vi "format_arcmin2arcsecstr.vi"(5 "RA arcmin":dbl, 9 "DEC Arcmin":dbl) -> (4 "Formatted RA":string, 8 "Formatted Dist":string, 15 "Formatted DEC":string)   [LabVIEW 2019]
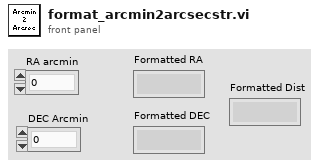
[diagram p1: front panel]
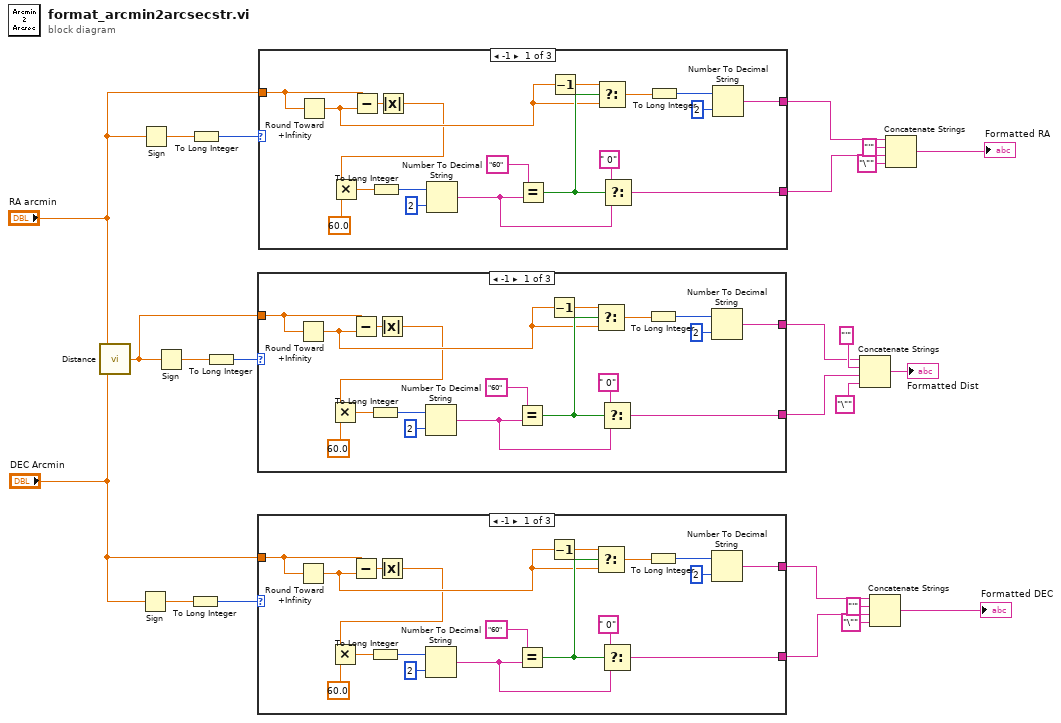
[diagram p0: block diagram]
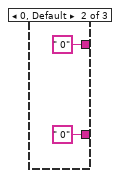
[diagram p2: hidden frame]
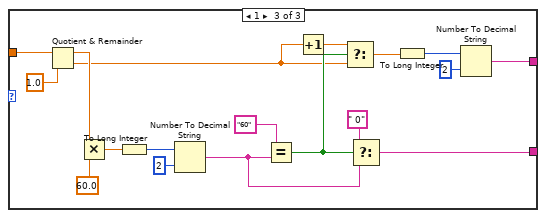
[diagram p3: hidden frame]
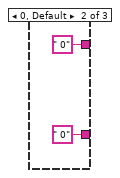
[diagram p4: hidden frame]
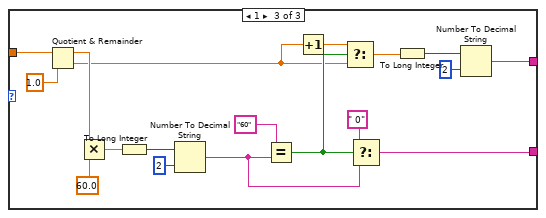
[diagram p5: hidden frame]
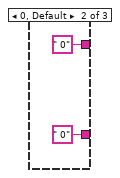
[diagram p6: hidden frame]
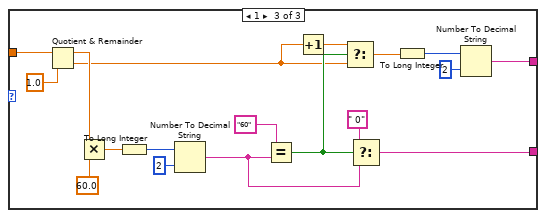
[diagram p7: hidden frame]
diagram:
  n1 = call "Distance.vi"("D2"="DEC Arcmin", "D1"="RA arcmin") -> ("DT"=w2:dbl)
  n2 = Sign(1:"DEC Arcmin") -> (0:w15:dbl)
  n3 = Sign(1:"RA arcmin") -> (0:w8:dbl)
  n4 = Sign(1:w2) -> (0:w9:dbl)
  n5 = To Long Integer(number=w15) -> (32bit integer=w14:i32)
  n6 = To Long Integer(number=w8) -> (32bit integer=w7:i32)
  n7 = To Long Integer(number=w9) -> (32bit integer=w10:i32)
  n8 = case shown="-1" w10 {
    tunnel: w2 -> [w28 _ w61]
    tunnel: [w29 " 0" w50] -> w6
    tunnel: [w30 " 0" w54] -> w5
    frame -1 {
      n9 = Round Toward +Infinity(x=w28) -> (ceil(x): smallest int >= x=w26:dbl)
      n10 = Subtract(x=w28, y=w26) -> (x-y=w27:dbl)
      n11 = Absolute Value(x=w27) -> (abs(x)=w25:dbl)
      n12 = Multiply(x=w25, y=60.0) -> (x*y=w40:dbl)
      n13 = To Long Integer(number=w40) -> (32bit integer=w42:i32)
      n14 = Number To Decimal String(number=w42, width (-)=i16 2) -> (decimal integer string=w35:string)
      n15 = Equal?(x="60", y=w35) -> (x = y?=w32:bool)
      n16 = Decrement(x=w26) -> (x-1=w33:dbl)
      n17 = Select(t=w33, s=w32, f=w26) -> (s? t:f=w31:dbl)
      n18 = Select(t=" 0", s=w32, f=w35) -> (s? t:f=w29:string)
      n19 = To Long Integer(number=w31) -> (32bit integer=w38:i32)
      n20 = Number To Decimal String(number=w38, width (-)=i16 2) -> (decimal integer string=w30:string)
    }
    frame 0, Default {
    }
    frame 1 {
      n21 = Quotient & Remainder(x=w61, y=1.0) -> (x-y*floor(x/y)=w48:dbl, floor(x/y)=w45:dbl)
      n22 = Multiply(x=w48, y=60.0) -> (x*y=w58:dbl)
      n23 = To Long Integer(number=w58) -> (32bit integer=w60:i32)
      n24 = Number To Decimal String(number=w60, width (-)=i16 2) -> (decimal integer string=w52:string)
      n25 = Equal?(x="60", y=w52) -> (x = y?=w47:bool)
      n26 = Increment(x=w45) -> (x+1=w49:dbl)
      n27 = Select(t=w49, s=w47, f=w45) -> (s? t:f=w46:dbl)
      n28 = Select(t=" 0", s=w47, f=w52) -> (s? t:f=w50:string)
      n29 = To Long Integer(number=w46) -> (32bit integer=w56:i32)
      n30 = Number To Decimal String(number=w56, width (-)=i16 2) -> (decimal integer string=w54:string)
    }
  }
  n31 = case shown="-1" w14 {
    tunnel: "DEC Arcmin" -> [w66 _ w99]
    tunnel: [w67 " 0" w88] -> w13
    tunnel: [w68 " 0" w92] -> w12
    frame -1 {
      n32 = Round Toward +Infinity(x=w66) -> (ceil(x): smallest int >= x=w64:dbl)
      n33 = Subtract(x=w66, y=w64) -> (x-y=w65:dbl)
      n34 = Absolute Value(x=w65) -> (abs(x)=w63:dbl)
      n35 = Multiply(x=w63, y=60.0) -> (x*y=w78:dbl)
      n36 = To Long Integer(number=w78) -> (32bit integer=w80:i32)
      n37 = Number To Decimal String(number=w80, width (-)=i16 2) -> (decimal integer string=w73:string)
      n38 = Equal?(x="60", y=w73) -> (x = y?=w70:bool)
      n39 = Decrement(x=w64) -> (x-1=w71:dbl)
      n40 = Select(t=w71, s=w70, f=w64) -> (s? t:f=w69:dbl)
      n41 = Select(t=" 0", s=w70, f=w73) -> (s? t:f=w67:string)
      n42 = To Long Integer(number=w69) -> (32bit integer=w76:i32)
      n43 = Number To Decimal String(number=w76, width (-)=i16 2) -> (decimal integer string=w68:string)
    }
    frame 0, Default {
    }
    frame 1 {
      n44 = Quotient & Remainder(x=w99, y=1.0) -> (x-y*floor(x/y)=w86:dbl, floor(x/y)=w83:dbl)
      n45 = Multiply(x=w86, y=60.0) -> (x*y=w96:dbl)
      n46 = To Long Integer(number=w96) -> (32bit integer=w98:i32)
      n47 = Number To Decimal String(number=w98, width (-)=i16 2) -> (decimal integer string=w90:string)
      n48 = Equal?(x="60", y=w90) -> (x = y?=w85:bool)
      n49 = Increment(x=w83) -> (x+1=w87:dbl)
      n50 = Select(t=w87, s=w85, f=w83) -> (s? t:f=w84:dbl)
      n51 = Select(t=" 0", s=w85, f=w90) -> (s? t:f=w88:string)
      n52 = To Long Integer(number=w84) -> (32bit integer=w94:i32)
      n53 = Number To Decimal String(number=w94, width (-)=i16 2) -> (decimal integer string=w92:string)
    }
  }
  n54 = case shown="-1" w7 {
    tunnel: "RA arcmin" -> [w104 _ w137]
    tunnel: [w105 " 0" w126] -> w4
    tunnel: [w106 " 0" w130] -> w3
    frame -1 {
      n55 = Round Toward +Infinity(x=w104) -> (ceil(x): smallest int >= x=w102:dbl)
      n56 = Subtract(x=w104, y=w102) -> (x-y=w103:dbl)
      n57 = Absolute Value(x=w103) -> (abs(x)=w101:dbl)
      n58 = Multiply(x=w101, y=60.0) -> (x*y=w116:dbl)
      n59 = To Long Integer(number=w116) -> (32bit integer=w118:i32)
      n60 = Number To Decimal String(number=w118, width (-)=i16 2) -> (decimal integer string=w111:string)
      n61 = Equal?(x="60", y=w111) -> (x = y?=w108:bool)
      n62 = Decrement(x=w102) -> (x-1=w109:dbl)
      n63 = Select(t=w109, s=w108, f=w102) -> (s? t:f=w107:dbl)
      n64 = Select(t=" 0", s=w108, f=w111) -> (s? t:f=w105:string)
      n65 = To Long Integer(number=w107) -> (32bit integer=w114:i32)
      n66 = Number To Decimal String(number=w114, width (-)=i16 2) -> (decimal integer string=w106:string)
    }
    frame 0, Default {
    }
    frame 1 {
      n67 = Quotient & Remainder(x=w137, y=1.0) -> (x-y*floor(x/y)=w124:dbl, floor(x/y)=w121:dbl)
      n68 = Multiply(x=w124, y=60.0) -> (x*y=w134:dbl)
      n69 = To Long Integer(number=w134) -> (32bit integer=w136:i32)
      n70 = Number To Decimal String(number=w136, width (-)=i16 2) -> (decimal integer string=w128:string)
      n71 = Equal?(x="60", y=w128) -> (x = y?=w123:bool)
      n72 = Increment(x=w121) -> (x+1=w125:dbl)
      n73 = Select(t=w125, s=w123, f=w121) -> (s? t:f=w122:dbl)
      n74 = Select(t=" 0", s=w123, f=w128) -> (s? t:f=w126:string)
      n75 = To Long Integer(number=w122) -> (32bit integer=w132:i32)
      n76 = Number To Decimal String(number=w132, width (-)=i16 2) -> (decimal integer string=w130:string)
    }
  }
  n77 = Concatenate Strings(w5, "'" ("string"), w6, "\"" ("string")) -> (→"Formatted Dist":string)
  n78 = Concatenate Strings(w12, "'" ("string"), w13, "\"" ("string")) -> (→"Formatted DEC":string)
  n79 = Concatenate Strings(w3, "'" ("string"), w4, "\"" ("string")) -> (→"Formatted RA":string)
